vi "Unsubscribe.vi"(8 "error in (no error)":errorcluster, 9 "Message ID":u16=10 format="%x", 10 "Topics To Unsubscribe From":string[](array[string]), 11 "connection ID":refnum<k5>) -> (0 "error out":errorcluster, 2 "Unsubscribe Message":u8[](array[numeric]) format="%x", 3 "connection ID out":refnum<k5>)   [LabVIEW 2020, in "DAQIO MQTT.lvlib"]
doc: "This VI unsubscribes the client from a topic. The client can no longer read published messages for the topic. \n\n© 2015 - daq.io, LLC - Peter Adelhardt"
uses:
  DAQIO MQTT.lvlib
  Controls/MessageType.ctl
  Controls/Retain_Flag.ctl
  Controls/DUP Flag.ctl
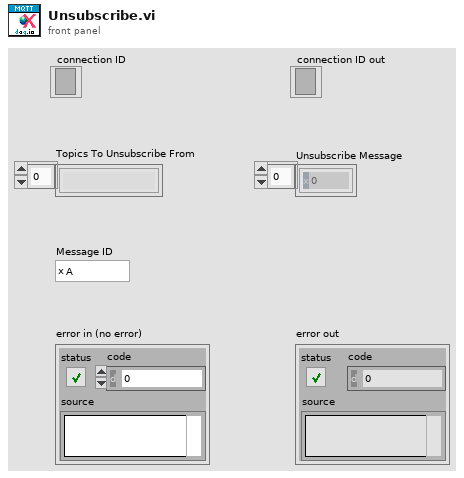
[diagram p1: front panel]
types:
  T1 = enum8{"At most once", "At least once", "Exactly once", "Reserved"}
  T2 = typedef "DAQIO MQTT.lvlib/DUP Flag.ctl" = bool
  T3 = typedef "DAQIO MQTT.lvlib/Retain_Flag.ctl" = bool
  T4 = typedef "DAQIO MQTT.lvlib/MessageType.ctl" = enum32{"Reserved", "CONNECT", "CONNACK", "PUBLISH", "PUBACK", "PUBREC", "PUBREL", "PUBCOMP", "SUBSCRIBE", "SUBACK", "UNSUBSCRIBE", "UNSUBACK", "PINGREQ", "PINGRESP", "DISCONNECT", "Reserved2"}
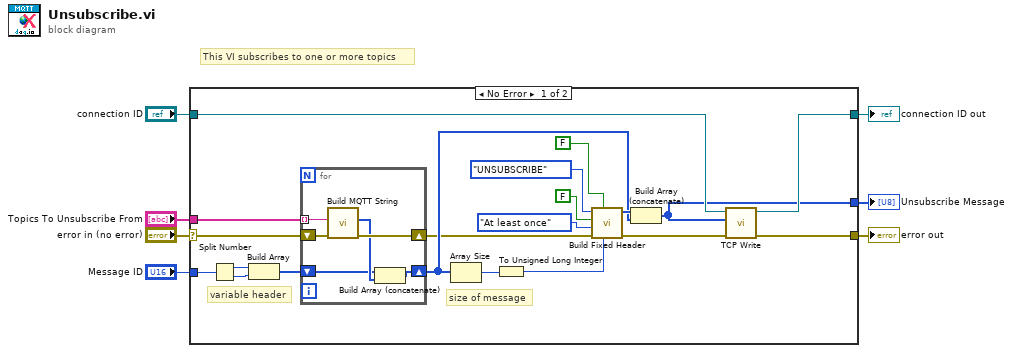
[diagram p0: block diagram]
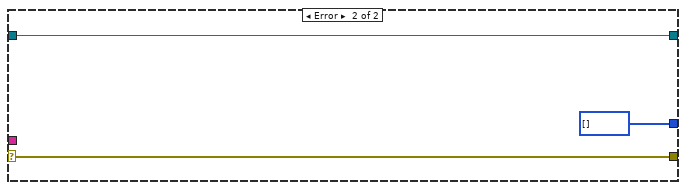
[diagram p2: hidden frame]
diagram:
  # "This VI subscribes to one or more topics"
  n1 = case shown="No Error" "error in (no error)" {
    selector: "error in (no error)" -> [w21 w36]
    tunnel: [w13 w36] -> w6
    tunnel: "Topics To Unsubscribe From" -> [w12 _]
    tunnel: "Message ID" -> [w11 _]
    tunnel: "connection ID" -> [w10 w35]
    tunnel: [w9 w35] -> w2
    tunnel: [w8 u8[] []] -> w1
    frame No Error {
      # "variable header"
      # "size of message"
      n2 = Split Number(x=w11) -> (hi(x)=w23:u8, lo(x)=w22:u8)
      n3 = Build Array(w23, w22) -> (w19:u8[])
      n4 = for {
        tunnel: w12 -> [w28] mode=indexing
        shift-right: [w32] -> w15
        shift-left: w21 -> [w33]
        shift-right: [w30] -> w20
        shift-left: w19 -> [w29]
        n5 = call "Build MQTT String.vi"("error in (no error)"=w33, "String to be encoded"=w28) -> ("error out"=w32:errorcluster, "UTF8 Byte Array"=w31:u8[])  [unwired: 8 in]
        n6 = Build Array (concatenate)(w29, w31) -> (w30:u8[])
      }
      n7 = Array Size(array=w20) -> (size(s)=w25:i32)
      n8 = To Unsigned Long Integer(number=w25) -> (unsigned 32bit integer=w26:u32)
      n9 = call "Build Fixed Header.vi"("Remaining Length"=w26, "Retain"=T3 FALSE, "error in (no error)"=w15, "QoS"=T1."At least once", "DUP"=T2 FALSE, "MessageType"=MessageType."UNSUBSCRIBE") -> ("error out"=w14:errorcluster, "Fixed Header"=w24:u8[])  [unwired: 4 in]
      n10 = Build Array (concatenate)(w24, w20) -> (w8:u8[])
      n11 = call "TCP Write.vi"("error in (no error)"=w14, "data in"=w8, "connection ID"=w10) -> ("error out"=w13:errorcluster, "connection ID out"=w9:refnum<k5>)  [unwired: 6 in, 1 out]
    }
    frame Error {
    }
  }
  "error out" <- w6
  "connection ID out" <- w2
  "Unsubscribe Message" <- w1
